vi "Parse Four Decimals.vi"(10 "Input String":string) -> (2 "Arg. Array":dbl[](array[numeric]))   [LabVIEW 2013]
doc: "This sub-VI parses four decimal numbers from a string with arguments of the form\n\"state:dec:dec:dec:dec\""
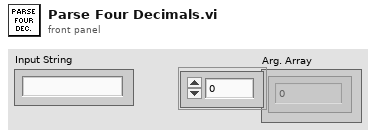
[diagram p1: front panel]
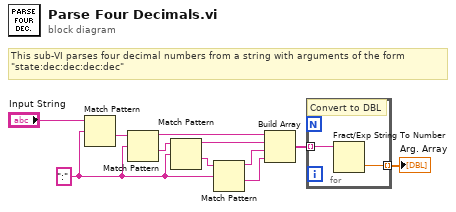
[diagram p0: block diagram]
diagram:
  w7 = ":" ("regular expression")
  # "This sub-VI parses four decimal numbers from a string with arguments of the form\n\"state:dec:dec:dec:dec\""
  n1 = Match Pattern(string="Input String", regular expression=w7) -> (after substring=w10:string)  [unwired: 1 in, 3 out]
  n2 = Match Pattern(string=w10, regular expression=w7) -> (before substring=w6:string, after substring=w9:string)  [unwired: 1 in, 2 out]
  n3 = Match Pattern(string=w9, regular expression=w7) -> (before substring=w5:string, after substring=w8:string)  [unwired: 1 in, 2 out]
  n4 = Match Pattern(string=w8, regular expression=w7) -> (before substring=w4:string, after substring=w3:string)  [unwired: 1 in, 2 out]
  n5 = Build Array(w6, w5, w4, w3) -> (w2:string[])
  n6 = for {
    tunnel: w2 -> [w13] mode=indexing
    tunnel: [w12] -> w1 mode=indexing
    # "Convert to DBL"
    n7 = Fract/Exp String To Number(string=w13) -> (number=w12:dbl)  [unwired: 3 in, 1 out]
  }
  "Arg. Array" <- w1
